vi "LvMPD_SimpleSimulator.vi"() -> ()   [LabVIEW 2012]
uses:
  <vilib>/Utility/error.llb/DialogType.ctl
  <vilib>/Utility/error.llb/whitespace.ctl
  <vilib>/regexp/Match Regular Expression.xnode
panel:
  out "Connect":bool
  out "Connected Client IP":string
  out "flag Exit":bool
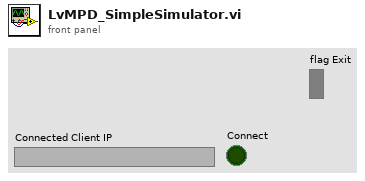
[diagram p1: front panel]
types:
  T1 = typedef "DialogType.ctl" = u16
  T2 = enum16{"Standard", "Buffered", "CRLF", "Immediate"}
  T3 = typedef "whitespace.ctl" = u16
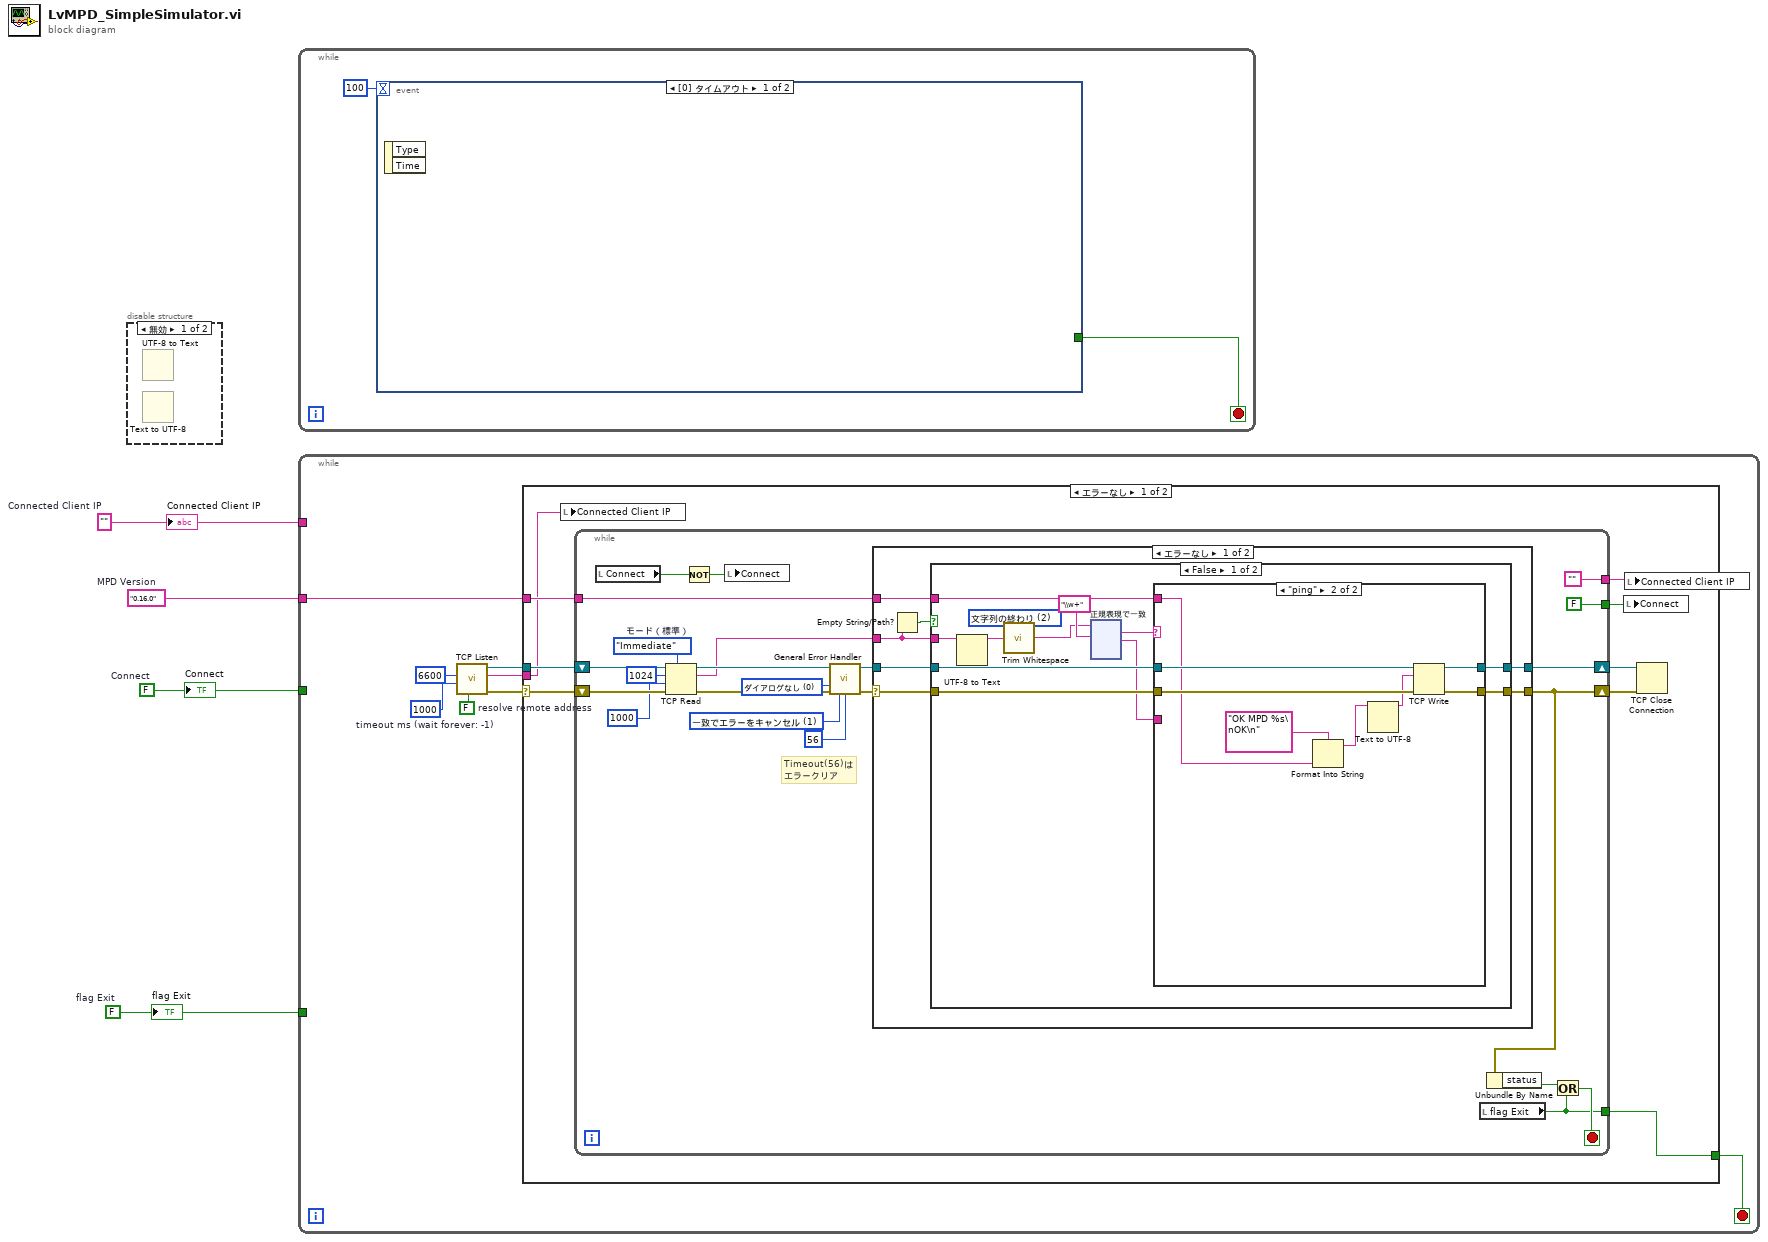
[diagram p0: block diagram]
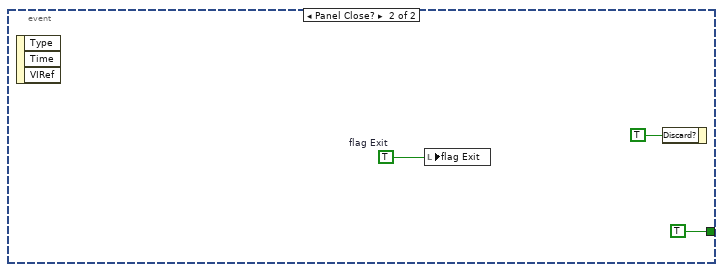
[diagram p3: hidden frame]
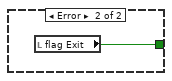
[diagram p7: hidden frame]
diagram:
  w1 = ""  # Connected Client IP
  w2 = FALSE  # Connect
  w3 = "0.16.0"  # MPD Version
  w4 = FALSE  # flag Exit
  n1 = disable-structure shown="無効" {
    frame Disabled {
      n2 = UTF-8 to Text() -> ()  [unwired: 2 in, 2 out]
      n3 = Text to UTF-8() -> ()  [unwired: 2 in, 2 out]
    }
    frame Enabled {
    }
  }
  n4 = while {
    stop <- w5 stop-if-true
    n5 = event shown="[0] タイムアウト" {
      selector: _ -> [_ _]
      dyn-events: _ -> [_ _]
      timeout: 100 -> [_ _]
      tunnel: [_ TRUE] -> w5
      event Timeout {
        n6 = event-data() -> ()  [unwired: 1 in, 2 out]
      }
      event Panel Close? {
        w7 = TRUE  # flag Exit
        n7 = event-data() -> ()  [unwired: 1 in, 3 out]
        n8 = local write "flag Exit"(w7) -> ()
        n9 = event-data("Discard?"=TRUE) -> ()  [unwired: 1 in, 1 out]
      }
    }
  }
  n10 = while {
    tunnel: w4 -> [_]
    tunnel: w3 -> [w12]
    tunnel: w2 -> [_]
    tunnel: w1 -> [_]
    stop <- w13 stop-if-true
    w10 = 1000  # timeout ms (wait forever: -1)
    w14 = FALSE  # resolve remote address
    n11 = call <vilib>:"TCP Listen.vi"("resolve remote address (T)"=w14, "timeout ms (wait forever: -1)"=w10, "port"=u16 6600) -> ("error out"=w16:errorcluster, "remote address"=w11:string, "connection ID"=w15:refnum<k5>)  [unwired: 4 in, 2 out]
    n12 = case shown="エラーなし" w16 {
      selector: w16 -> [w24 _]
      tunnel: w15 -> [w26 _]
      tunnel: [w21 w193] -> w13
      tunnel: w12 -> [w22 _]
      tunnel: w11 -> [w18 _]
      frame No Error {
        n13 = local write "Connected Client IP"(w18) -> ()
        n14 = while {
          shift-right: [w47] -> w25
          shift-left: w26 -> [w48]
          shift-right: [w34] -> w23
          shift-left: w24 -> [w44]
          tunnel: w22 -> [w36]
          tunnel: [w32] -> w21
          tunnel: [FALSE] -> w20
          tunnel: [""] -> w19
          stop <- w35 stop-if-true
          w40 = 1 items=["例外なし", "一致でエラーをキャンセル", "一致でエラーをセット"] ("[exception action] (none:0)")
          w41 = T1 0 items=["ダイアログなし", "OKメッセージ", "継続か停止メッセージ", "OKメッセージ+警告", "継続/停止+警告"] ("type of dialog (OK msg:1)")
          w45 = T2."Immediate"  # モード（標準）
          # "Timeout(56)は\nエラークリア"
          n15 = local read "Connect"() -> (w30:bool)
          n16 = TCP Read(connection ID=w48, bytes to read=1024, error in (no error)=w44, 7:w45, 9:1000) -> (connection ID out=w46:refnum<k5>, data out=w42:string, error out=w38:errorcluster)
          n17 = Not(x=w30) -> (.not. x?=w29:bool)
          n18 = local write "Connect"(w29) -> ()
          n19 = call <vilib>:"General Error Handler.vi"("type of dialog (OK msg:1)"=w41, "error in (no error)"=w38, "[exception action] (none:0)"=w40, "[exception code]"=56) -> ("error out"=w37:errorcluster)  [unwired: 7 in, 4 out]
          n20 = case shown="エラーなし" w37 {
            selector: w37 -> [w53 w191]
            tunnel: [w49 w192] -> w47
            tunnel: w46 -> [w55 w192]
            tunnel: w42 -> [w50 _]
            tunnel: [w54 w191] -> w34
            tunnel: w36 -> [w52 _]
            frame No Error {
              n21 = Empty String/Path?(string/path=w50) -> (empty?=w51:bool)
              n22 = case shown="FALSE" w51 {
                tunnel: w55 -> [w66 w190]
                tunnel: [w65 w189] -> w54
                tunnel: w53 -> [w64 w189]
                tunnel: w52 -> [w62 _]
                tunnel: w50 -> [w61 _]
                tunnel: [w67 w190] -> w49
                frame False {
                  w63 = T3 2 items=["両方", "文字列の先頭", "文字列の終わり"] ("location (both)")
                  n23 = UTF-8 to Text(11:w61) -> (3:w60:string)  [unwired: 1 in, 1 out]
                  n24 = call <vilib>:"Trim Whitespace.vi"("string"=w60, "location (both)"=w63) -> ("trimmed string"=w57:string)
                  n25 = xnode "正規表現で一致"("入力文字列"=w57, "正規表現"="\\w+" ("入力文字列")) -> ("全体一致"=w59:string, "一致の後"=w56:string)  [unwired: 4 in, 3 out]
                  n26 = case shown="\"ping\"" w59 {
                    tunnel: [w180 w188] -> w67
                    tunnel: w66 -> [w180 w187]
                    tunnel: [w179 w186] -> w65
                    tunnel: w64 -> [w179 w185]
                    tunnel: w62 -> [_ w184]
                    tunnel: w56 -> [_ _]
                    frame Default {
                      # "#エラー応答"
                      # "\"OK MPD 0.16.0\nACK [5@0] {} unknown command \"lsfiles\"\""
                    }
                    frame "ping" {
                      n27 = Format Into String(format string="OK MPD %s\nOK\n", w184) -> (resulting string=w183:string)  [unwired: 2 in, 1 out]
                      n28 = Text to UTF-8(11:w183) -> (3:w181:string)  [unwired: 1 in, 1 out]
                      n29 = TCP Write(connection ID=w187, data in=w181, error in (no error)=w185) -> (connection ID out=w188:refnum<k5>, error out=w186:errorcluster)  [unwired: 1 in, 1 out]
                    }
                  }
                }
                frame True {
                }
              }
            }
            frame Error {
            }
          }
          n30 = local read "flag Exit"() -> (w32:bool)
          n31 = Unbundle By Name(w34) -> ("status"=w33:bool)
          n32 = Or(x=w33, y=w32) -> (x .or. y?=w35:bool)
        }
        n33 = local write "Connect"(w20) -> ()
        n34 = local write "Connected Client IP"(w19) -> ()
        n35 = TCP Close Connection(connection ID=w25, error in (no error)=w23) -> ()  [unwired: 1 in, 2 out]
      }
      frame Error {
        n36 = local read "flag Exit"() -> (w193:bool)
      }
    }
  }
  "flag Exit" <- w4
  "Connect" <- w2
  "Connected Client IP" <- w1
